vi "Render.vi"(8 "error in (no error)":errorcluster) -> (0 "error out":errorcluster)   [LabVIEW 2018, in "Markdown.lvlib"]
doc: "Render the Library markdown."
uses:
  Markdown.lvlib
  Global.vi
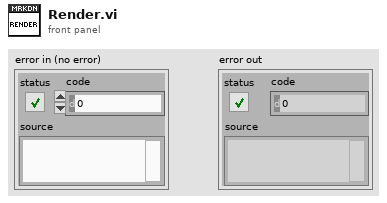
[diagram p1: front panel]
types:
  T1 = typedef "Markdown.lvlib/Item.ctl" = cluster{"Name":string, "Icon":picture, "Path":path, "Title":string, "Desc":string, "ConPane":picture, "TypeString":string, "ProjectItem":string, "VI Type":enum32{"invalid VI type", "Standard VI", "Control VI", "Global VI", "Polymorphic VI", "Configuration VI", "SubSystem", "Facade VI", "Method VI", "Statechart Diagram VI"}}
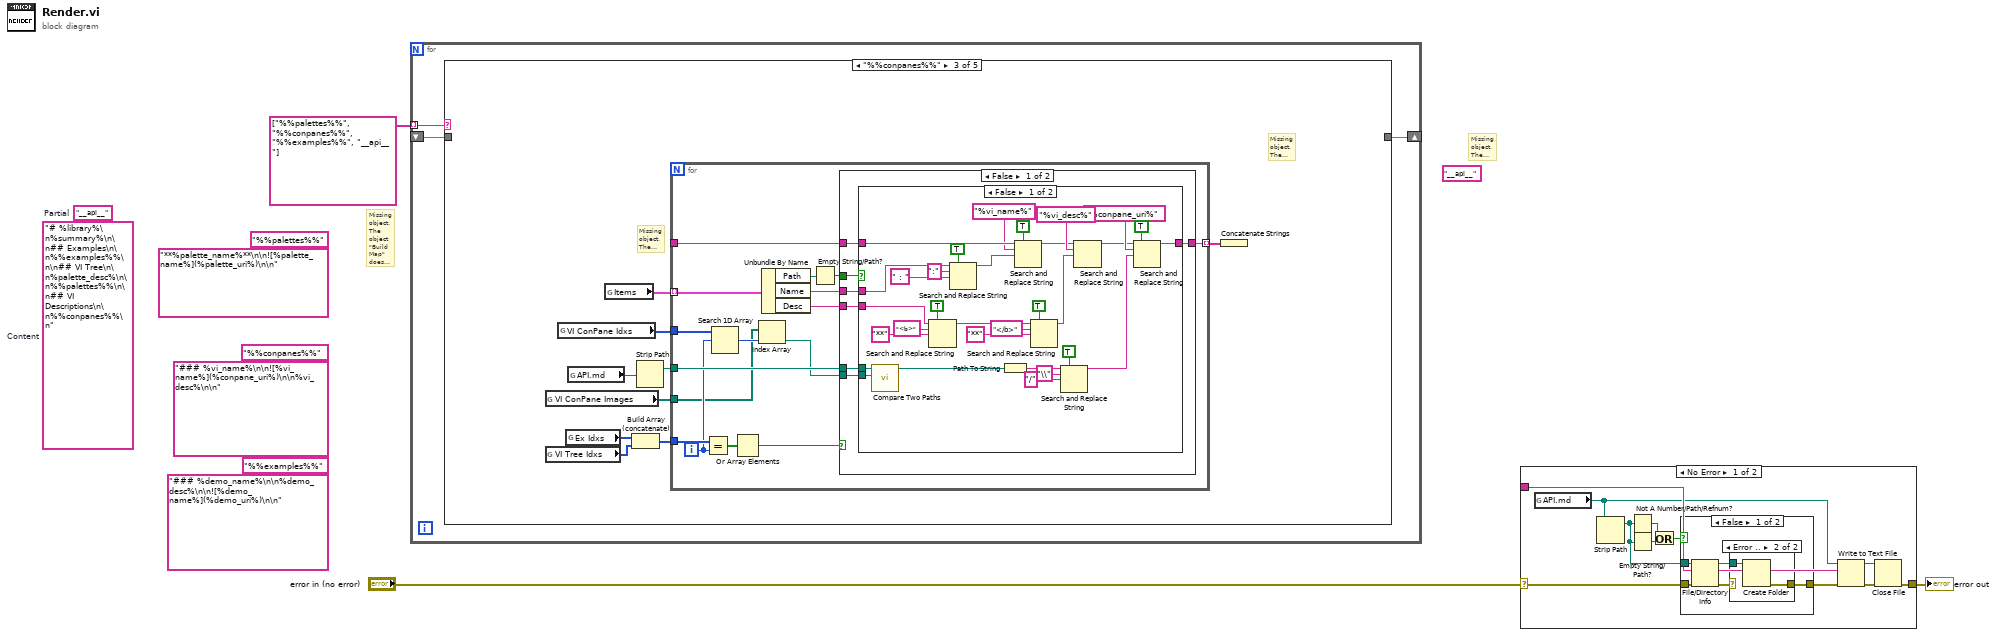
[diagram p0: block diagram]
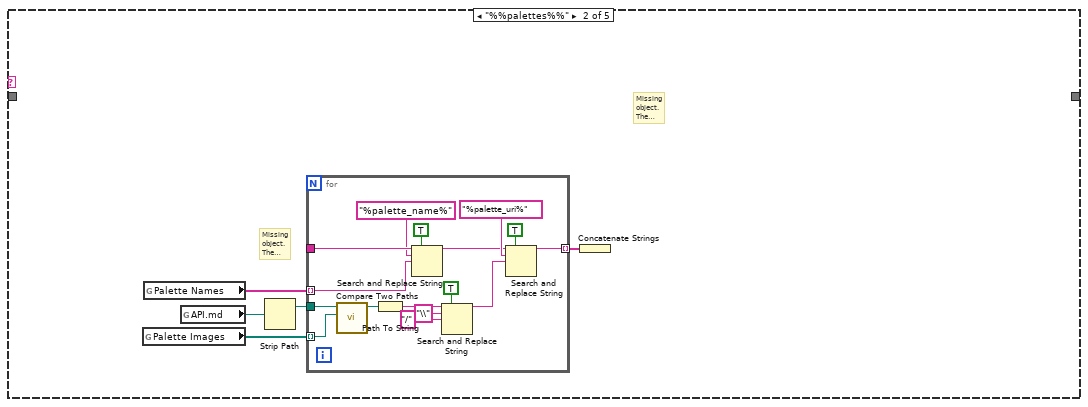
[diagram p6: hidden frame]
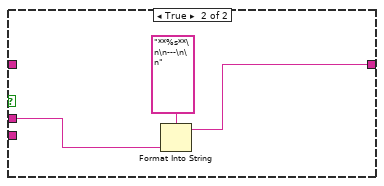
[diagram p7: hidden frame]
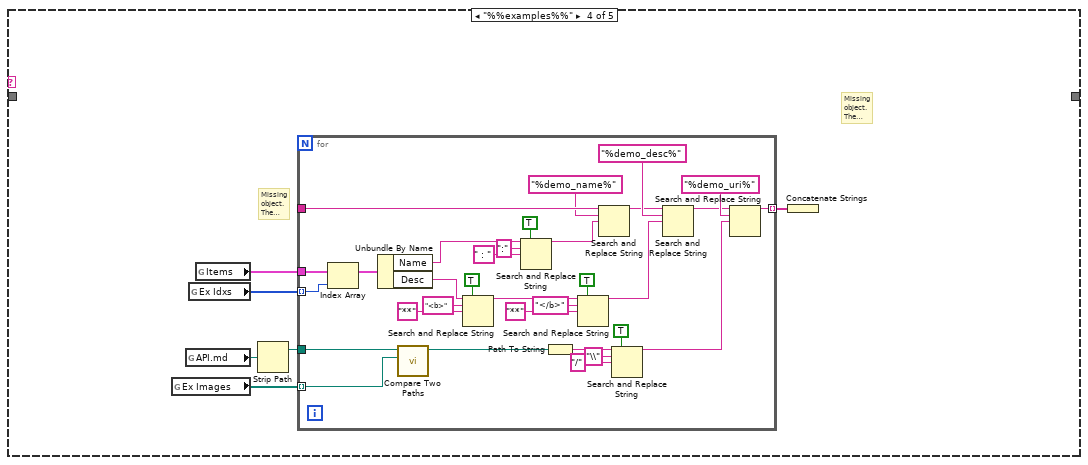
[diagram p9: hidden frame]
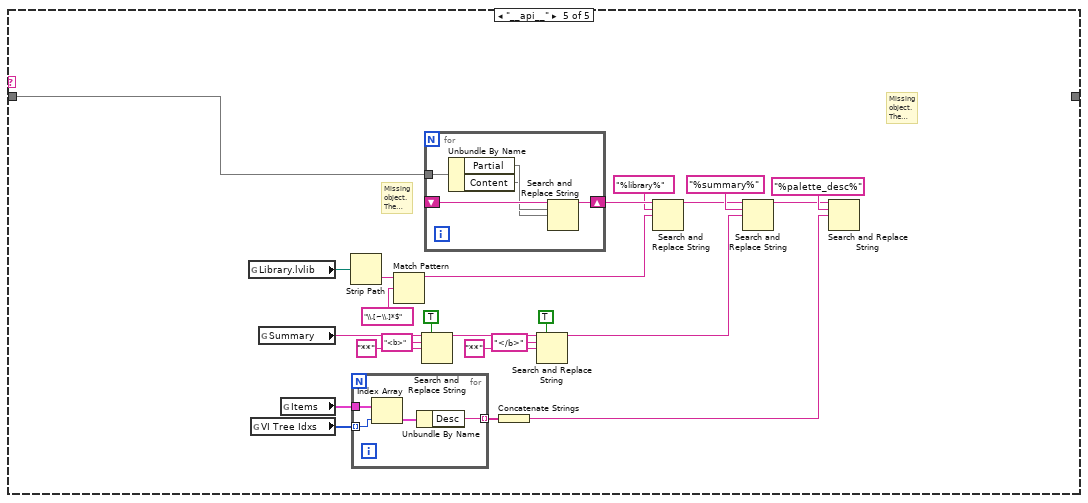
[diagram p10: hidden frame]
diagram:
  w3 = "__api__" ("key")
  w6 = "%%examples%%"
  w5 = "### %demo_name%\n\n%demo_desc%\n\n![%demo_name%](%demo_uri%)\n\n"
  w8 = "%%conpanes%%"
  w7 = "### %vi_name%\n\n![%vi_name%](%conpane_uri%)\n\n%vi_desc%\n\n"
  w12 = "__api__"  # Partial
  w10 = "%%palettes%%"
  w9 = "**%palette_name%**\n\n![%palette_name%](%palette_uri%)\n\n"
  w11 = "# %library%\n%summary%\n\n## Examples\n\n%%examples%%\n\n## VI Tree\n\n%palette_desc%\n\n%%palettes%%\n\n## VI Descriptions\n\n%%conpanes%%\n"  # Content
  # "Missing object. The object \"Look In Map\" does not exist in the previous version."
  # "Missing object. The object \"Build Map\" does not exist in the previous version."
  n1 = for {
    tunnel: string[] ["%%palettes%%", "%%conpanes%%", "%%examples%%", "__api__"] -> [w18] mode=indexing
    shift-right: [w16] -> w2
    shift-left: [w17] -> w4
    n2 = case shown="\"%%conpanes%%\"" w18 {
      selector: w18 -> [_ w25 w53 w121 w168]
      tunnel: w17 -> [w19 w24 w52 w120 w162]
      tunnel: [w19 w23 w51 w119 w161] -> w16
      frame Default {
      }
      frame "%%palettes%%" {
        # "Missing object. The object \"Look In Map\" does not exist in the previous version."
        # "Missing object. The object \"Insert Into Map\" does not exist in the previous version."
        n3 = global read "Global.vi" "Palette Images"() -> (w20:path[])
        n4 = global read "Global.vi" "Palette Names"() -> (w22:string[])
        n5 = global read "Global.vi" "API.md"() -> (w21:path)
        n6 = Strip Path(path=w21) -> (stripped path=w26:path)  [unwired: 1 out]
        n7 = for {
          tunnel: _ -> [w44]
          tunnel: w22 -> [w29] mode=indexing
          tunnel: w26 -> [w42]
          tunnel: w20 -> [w41] mode=indexing
          tunnel: [w37] -> w28 mode=indexing
          n8 = call <vilib>:"Compare Two Paths.vi"("Path 2"=w41, "Path 1"=w42) -> ("Relative Path from 1 to 2"=w38:path)  [unwired: 6 in, 3 out]
          n9 = Path To String(path=w38) -> (string=w35:string)
          n10 = Search and Replace String(replace all?=TRUE ("replace all? (F)"), input string=w44, search string="%palette_name%", replace string=w29) -> (result string=w39:string)  [unwired: 4 in, 3 out]
          n11 = Search and Replace String(replace all?=TRUE ("replace all? (F)"), input string=w35, search string="\\", replace string="/" ("search string")) -> (result string=w32:string)  [unwired: 4 in, 3 out]
          n12 = Search and Replace String(replace all?=TRUE ("replace all? (F)"), input string=w39, search string="%palette_uri%", replace string=w32) -> (result string=w37:string)  [unwired: 4 in, 3 out]
        }
        n13 = Concatenate Strings(w28) -> (w27:string)
      }
      frame "%%conpanes%%" {
        # "Missing object. The object \"Look In Map\" does not exist in the previous version."
        # "Missing object. The object \"Insert Into Map\" does not exist in the previous version."
        n14 = global read "Global.vi" "VI ConPane Images"() -> (w47:path[])
        n15 = global read "Global.vi" "VI Tree Idxs"() -> (w45:i32[])
        n16 = global read "Global.vi" "VI ConPane Idxs"() -> (w49:i32[])
        n17 = global read "Global.vi" "Ex Idxs"() -> (w46:i32[])
        n18 = global read "Global.vi" "API.md"() -> (w48:path)
        n19 = global read "Global.vi" "Items"() -> (w50:T1[])
        n20 = Build Array (concatenate)(w46, w45) -> (w57:i32[])
        n21 = Strip Path(path=w48) -> (stripped path=w56:path)  [unwired: 1 out]
        n22 = for {
          tunnel: _ -> [w73]
          tunnel: w50 -> [w63] mode=indexing
          tunnel: w56 -> [w71]
          tunnel: w47 -> [w58]
          tunnel: [w70] -> w54 mode=indexing
          tunnel: w57 -> [w66]
          tunnel: w49 -> [w62]
          i -> [w61]
          n23 = Equal?(x=w66, y=w61) -> (x = y?=w65:bool[])
          n24 = Search 1D Array(1D array=w62, element=w61) -> (index of element=w60:i32)  [unwired: 1 in]
          n25 = Or Array Elements(Boolean array=w65) -> (logical OR=w64:bool)
          n26 = Index Array(array=w58, index=w60) -> (element=w59:path)
          n27 = Unbundle By Name(w63) -> ("Path"=w68:path, "Name"=w72:string, "Desc"=w69:string)
          n28 = Empty String/Path?(string/path=w68) -> (empty?=w67:bool)
          n29 = case shown="False" w64 {
            tunnel: w73 -> [w80 _]
            tunnel: w72 -> [w79 _]
            tunnel: w71 -> [w78 _]
            tunnel: w59 -> [w77 _]
            tunnel: [w76 _] -> w70
            tunnel: w69 -> [w75 _]
            tunnel: w67 -> [w74 _]
            frame False {
              n30 = case shown="False" w74 {
                tunnel: w80 -> [w111 _]
                tunnel: w79 -> [w84 w114]
                tunnel: w78 -> [w109 _]
                tunnel: w77 -> [w108 _]
                tunnel: [w106 w113] -> w76
                tunnel: w75 -> [w101 _]
                frame False {
                  n31 = call <vilib>:"Compare Two Paths.vi"("Path 2"=w108, "Path 1"=w109) -> ("Relative Path from 1 to 2"=w89:path)  [unwired: 6 in, 3 out]
                  n32 = Search and Replace String(replace all?=TRUE ("replace all? (F)"), input string=w101, search string="<b>", replace string="**" ("replace string (\"\")")) -> (result string=w95:string)  [unwired: 4 in, 3 out]
                  n33 = Search and Replace String(replace all?=TRUE ("replace all? (F)"), input string=w84, search string=":", replace string=" : " ("replace string (\"\")")) -> (result string=w83:string)  [unwired: 4 in, 3 out]
                  n34 = Path To String(path=w89) -> (string=w92:string)
                  n35 = Search and Replace String(replace all?=TRUE ("replace all? (F)"), input string=w111, search string="%vi_name%", replace string=w83) -> (result string=w104:string)  [unwired: 4 in, 3 out]
                  n36 = Search and Replace String(replace all?=TRUE ("replace all? (F)"), input string=w95, search string="</b>", replace string="**" ("replace string (\"\")")) -> (result string=w94:string)  [unwired: 4 in, 3 out]
                  n37 = Search and Replace String(replace all?=TRUE ("replace all? (F)"), input string=w92, search string="\\", replace string="/" ("search string")) -> (result string=w88:string)  [unwired: 4 in, 3 out]
                  n38 = Search and Replace String(input string=w104, search string="%vi_desc%", replace string=w94) -> (result string=w103:string)  [unwired: 5 in, 3 out]
                  n39 = Search and Replace String(replace all?=TRUE ("replace all? (F)"), input string=w103, search string="%conpane_uri%", replace string=w88) -> (result string=w106:string)  [unwired: 4 in, 3 out]
                }
                frame True {
                  n40 = Format Into String(format string="**%s**\n\n---\n\n" ("result string"), w114) -> (resulting string=w113:string)  [unwired: 2 in, 1 out]
                }
              }
            }
            frame True {
              # "Ignore Example and VI Tree VIs"
            }
          }
        }
        n41 = Concatenate Strings(w54) -> (w55:string)
      }
      frame "%%examples%%" {
        # "Missing object. The object \"Look In Map\" does not exist in the previous version."
        # "Missing object. The object \"Insert Into Map\" does not exist in the previous version."
        n42 = global read "Global.vi" "Ex Images"() -> (w115:path[])
        n43 = global read "Global.vi" "API.md"() -> (w116:path)
        n44 = global read "Global.vi" "Ex Idxs"() -> (w117:i32[])
        n45 = global read "Global.vi" "Items"() -> (w118:T1[])
        n46 = Strip Path(path=w116) -> (stripped path=w122:path)  [unwired: 1 out]
        n47 = for {
          tunnel: _ -> [w156]
          tunnel: w118 -> [w154]
          tunnel: w122 -> [w153]
          tunnel: w115 -> [w152] mode=indexing
          tunnel: [w150] -> w124 mode=indexing
          tunnel: w117 -> [w130] mode=indexing
          n48 = Index Array(array=w154, index=w130) -> (element=w131:T1)
          n49 = Unbundle By Name(w131) -> ("Name"=w126:string, "Desc"=w145:string)
          n50 = call <vilib>:"Compare Two Paths.vi"("Path 2"=w152, "Path 1"=w153) -> ("Relative Path from 1 to 2"=w133:path)  [unwired: 6 in, 3 out]
          n51 = Search and Replace String(replace all?=TRUE ("replace all? (F)"), input string=w145, search string="<b>", replace string="**" ("replace string (\"\")")) -> (result string=w139:string)  [unwired: 4 in, 3 out]
          n52 = Search and Replace String(replace all?=TRUE ("replace all? (F)"), input string=w126, search string=":", replace string=" : " ("replace string (\"\")")) -> (result string=w125:string)  [unwired: 4 in, 3 out]
          n53 = Path To String(path=w133) -> (string=w136:string)
          n54 = Search and Replace String(replace all?=TRUE ("replace all? (F)"), input string=w139, search string="</b>", replace string="**" ("replace string (\"\")")) -> (result string=w138:string)  [unwired: 4 in, 3 out]
          n55 = Search and Replace String(input string=w156, search string="%demo_name%", replace string=w125) -> (result string=w148:string)  [unwired: 5 in, 3 out]
          n56 = Search and Replace String(replace all?=TRUE ("replace all? (F)"), input string=w136, search string="\\", replace string="/" ("search string")) -> (result string=w132:string)  [unwired: 4 in, 3 out]
          n57 = Search and Replace String(input string=w148, search string="%demo_desc%", replace string=w138) -> (result string=w147:string)  [unwired: 5 in, 3 out]
          n58 = Search and Replace String(input string=w147, search string="%demo_uri%", replace string=w132) -> (result string=w150:string)  [unwired: 5 in, 3 out]
        }
        n59 = Concatenate Strings(w124) -> (w123:string)
      }
      frame "__api__" {
        # "Missing object. The object \"Insert Into Map\" does not exist in the previous version."
        # "Missing object. The object \"Look In Map\" does not exist in the previous version."
        n60 = global read "Global.vi" "Library.lvlib"() -> (w160:path)
        n61 = global read "Global.vi" "VI Tree Idxs"() -> (w157:i32[])
        n62 = global read "Global.vi" "Summary"() -> (w159:string)
        n63 = global read "Global.vi" "Items"() -> (w158:T1[])
        n64 = Strip Path(path=w160) -> (name=w180:string)  [unwired: 1 out]
        n65 = for {
          tunnel: w158 -> [w187]
          tunnel: w157 -> [w186] mode=indexing
          tunnel: [w184] -> w166 mode=indexing
          n66 = Index Array(array=w187, index=w186) -> (element=w185:T1)
          n67 = Unbundle By Name(w185) -> ("Desc"=w184:string)
        }
        n68 = Match Pattern(string=w180, regular expression="\\.[~\\.]*$") -> (before substring=w179:string)  [unwired: 4 out]
        n69 = Search and Replace String(replace all?=TRUE ("replace all? (F)"), input string=w159, search string="<b>", replace string="**" ("replace string (\"\")")) -> (result string=w170:string)  [unwired: 4 in, 3 out]
        n70 = for {
          tunnel: w162 -> [w192]
          shift-right: [w188] -> w183
          shift-left: _ -> [w191]
          n71 = Unbundle By Name(w192) -> ("Partial"=w190, "Content"=w189)
          n72 = Search and Replace String(input string=w191, search string=w190, replace string=w189) -> (result string=w188:string)  [unwired: 5 in, 3 out]
        }
        n73 = Concatenate Strings(w166) -> (w165:string)
        n74 = Search and Replace String(replace all?=TRUE ("replace all? (F)"), input string=w170, search string="</b>", replace string="**" ("replace string (\"\")")) -> (result string=w169:string)  [unwired: 4 in, 3 out]
        n75 = Search and Replace String(input string=w183, search string="%library%", replace string=w179) -> (result string=w177:string)  [unwired: 5 in, 3 out]
        n76 = Search and Replace String(input string=w177, search string="%summary%", replace string=w169) -> (result string=w164:string)  [unwired: 5 in, 3 out]
        n77 = Search and Replace String(input string=w164, search string="%palette_desc%", replace string=w165) -> (result string=w163:string)  [unwired: 5 in, 3 out]
      }
    }
  }
  n78 = case shown="No Error" "error in (no error)" {
    selector: "error in (no error)" -> [w196 w213]
    tunnel: [w195 w213] -> w13
    tunnel: [w194 _] -> w1
    frame No Error {
      n79 = global read "Global.vi" "API.md"() -> (w193:path)
      n80 = Strip Path(path=w193) -> (stripped path=w197:path)  [unwired: 1 out]
      n81 = Not A Number/Path/Refnum?(number/path/refnum=w197) -> (NaN/Path/Refnum?=w200:bool)
      n82 = Empty String/Path?(string/path=w197) -> (empty?=w201:bool)
      n83 = Or(x=w200, y=w201) -> (x .or. y?=w199:bool)
      n84 = case shown="False" w199 {
        tunnel: w196 -> [w208 w212]
        tunnel: [w206 w212] -> w198
        tunnel: w197 -> [w204 _]
        frame False {
          n85 = File/Directory Info(path=w204, error in=w208) -> (path out=w205:path, error out=w207:errorcluster)  [unwired: 5 out]
          n86 = case shown="Error .." w207 {
            selector: w207 -> [w209 _]
            tunnel: [w209 w211] -> w206
            tunnel: w205 -> [_ w210]
            frame No Error {
            }
            frame Error {
              n87 = Create Folder(path (use dialog)=w210) -> (error out=w211:errorcluster)  [unwired: 2 in, 2 out]
            }
          }
        }
        frame True {
        }
      }
      n88 = Write to Text File(file (use dialog)=w193, text=w194, error in=w198) -> (refnum out=w202:refnum<file>, error out=w203:errorcluster)  [unwired: 1 in, 1 out]
      n89 = Close File(refnum=w202, error in=w203) -> (error out=w195:errorcluster)  [unwired: 1 out]
    }
    frame Error {
    }
  }
  "error out" <- w13
